vi "Lab14_LabView.vi"() -> ()   [LabVIEW 2022 SP3]
uses:
  <vilib>/Instr/_visa.llb/VISA Configure Serial Port (Instr).vi
panel:
  out "POTENCIOMETRO 8":dbl(knob) scale=0.0..1023.0
  out "POTENCIOMETRO 7":dbl(knob) scale=0.0..1023.0
  out "POTENCIOMETRO 6":dbl(knob) scale=0.0..1023.0
  out "POTENCIOMETRO 5":dbl(knob) scale=0.0..1023.0
  out "POTENCIOMETRO 4":dbl(knob) scale=0.0..1023.0
  out "POTENCIOMETRO 3":dbl(knob) scale=0.0..1023.0
  out "POTENCIOMETRO 2":dbl(knob) scale=0.0..1023.0
  out "POTENCIOMETRO":i32(knob) scale=0.0..1023.0
  in  "VISA resource name":refnum<visa-resource-name>
  in  "stop":bool
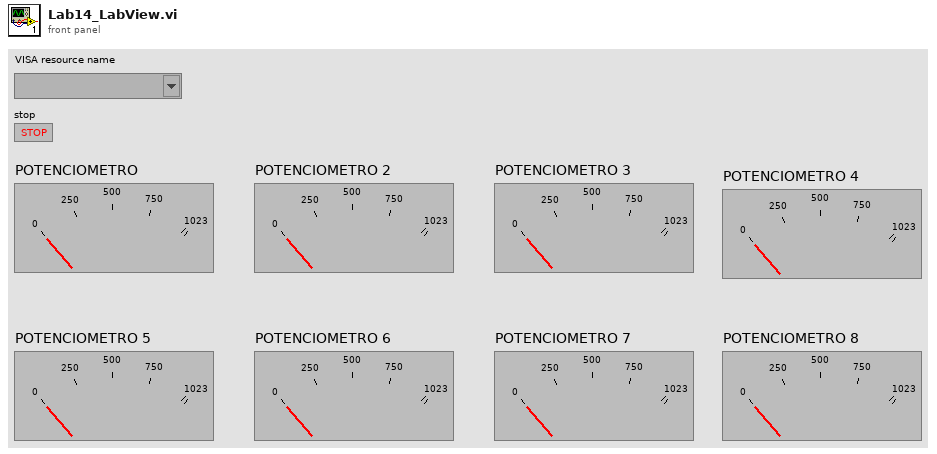
[diagram p1: front panel]
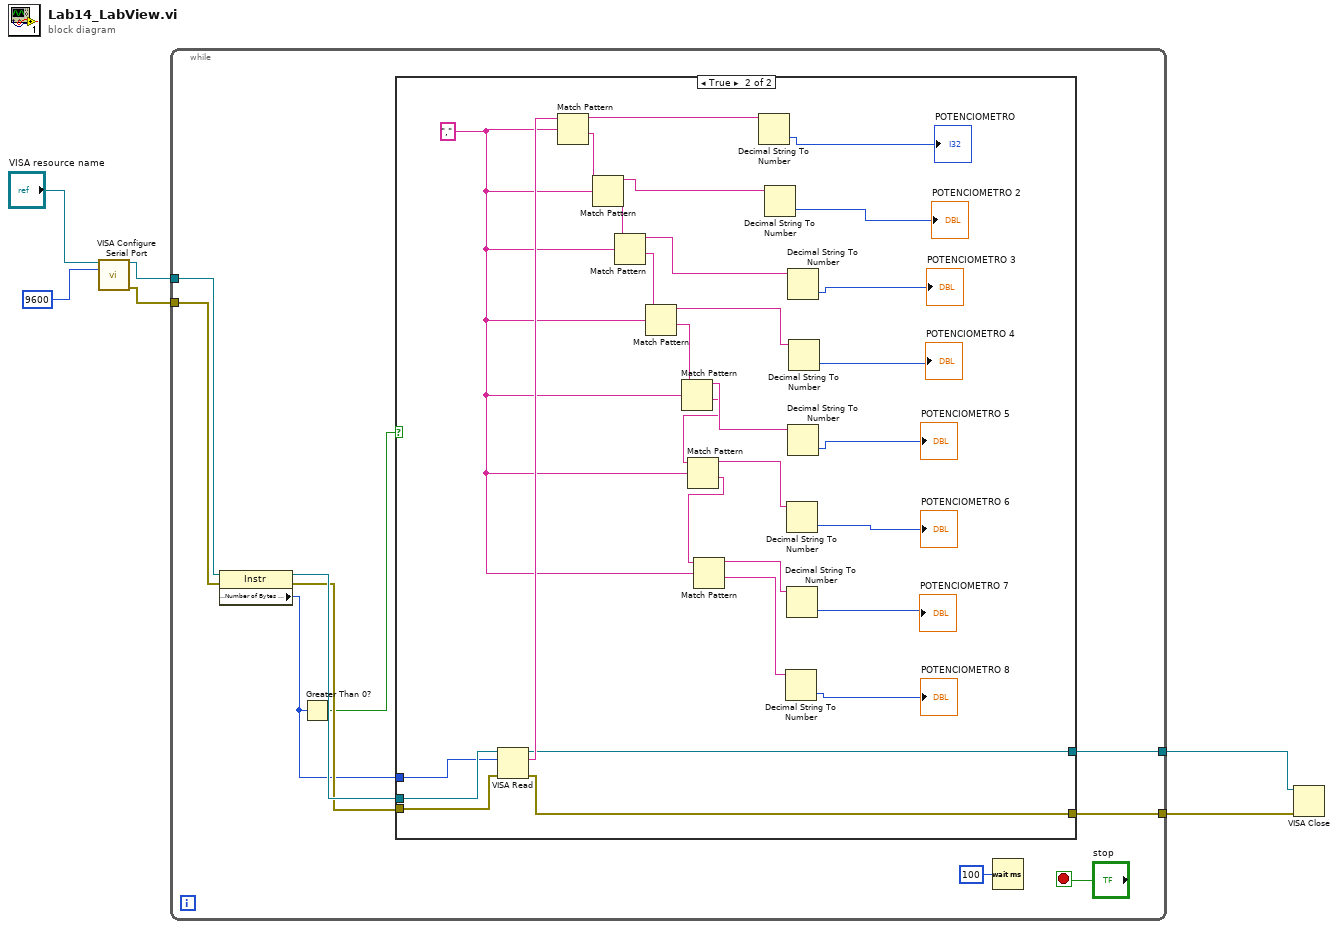
[diagram p0: block diagram]
diagram:
  n1 = call-poly "VISA Configure Serial Port"("VISA resource name"="VISA resource name", "baud rate (9600)"=u32 9600) -> ("VISA resource name out"=w6:refnum<visa-resource-name>, "error out"=w5:errorcluster)  [unwired: 12 in]
  n2 = while {
    tunnel: w6 -> [w10]
    tunnel: w5 -> [w9]
    tunnel: [w8] -> w2
    tunnel: [w7] -> w1
    stop <- "stop" stop-if-true
    n3 = property class="Instr"(reference=w10, error in=w9) -> (reference out=w14:refnum<visa-resource-name>, error out=w13:errorcluster, "Serial Settings:Number of Bytes at Serial Port"=w11:u32)
    n4 = Greater Than 0?(x=w11) -> (x > 0?=w12:bool)
    n5 = case shown="True" w12 {
      tunnel: w14 -> [w18 w47]
      tunnel: w13 -> [w17 w46]
      tunnel: w11 -> [_ w45]
      tunnel: [w17 w20] -> w8
      tunnel: [w18 w19] -> w7
      frame False {
      }
      frame True {
        w26 = ","
        n6 = VISA Read(VISA resource name=w47, byte count=w45, error in (no error)=w46) -> (VISA resource name out=w19:refnum<visa-resource-name>, read buffer=w44:string, error out=w20:errorcluster)  [unwired: 1 out]
        n7 = Match Pattern(string=w44, regular expression=w26) -> (before substring=w43:string, after substring=w42:string)  [unwired: 1 in, 2 out]
        n8 = Match Pattern(string=w42, regular expression=w26) -> (before substring=w41:string, after substring=w40:string)  [unwired: 1 in, 2 out]
        n9 = Match Pattern(string=w40, regular expression=w26) -> (before substring=w39:string, after substring=w38:string)  [unwired: 1 in, 2 out]
        n10 = Match Pattern(string=w38, regular expression=w26) -> (before substring=w36:string, after substring=w37:string)  [unwired: 1 in, 2 out]
        n11 = Match Pattern(string=w37, regular expression=w26) -> (before substring=w35:string, after substring=w25:string)  [unwired: 1 in, 2 out]
        n12 = Match Pattern(string=w25, regular expression=w26) -> (before substring=w23:string, after substring=w24:string)  [unwired: 1 in, 2 out]
        n13 = Match Pattern(string=w24, regular expression=w26) -> (before substring=w22:string, after substring=w21:string)  [unwired: 1 in, 2 out]
        n14 = Decimal String To Number(string=w43) -> (number=→"POTENCIOMETRO":i32)  [unwired: 2 in, 1 out]
        n15 = Decimal String To Number(string=w41) -> (number=→"POTENCIOMETRO 2":i32)  [unwired: 2 in, 1 out]
        n16 = Decimal String To Number(string=w21) -> (number=→"POTENCIOMETRO 8":i32)  [unwired: 2 in, 1 out]
        n17 = Decimal String To Number(string=w23) -> (number=→"POTENCIOMETRO 6":i32)  [unwired: 2 in, 1 out]
        n18 = Decimal String To Number(string=w22) -> (number=→"POTENCIOMETRO 7":i32)  [unwired: 2 in, 1 out]
        n19 = Decimal String To Number(string=w39) -> (number=→"POTENCIOMETRO 3":i32)  [unwired: 2 in, 1 out]
        n20 = Decimal String To Number(string=w35) -> (number=→"POTENCIOMETRO 5":i32)  [unwired: 2 in, 1 out]
        n21 = Decimal String To Number(string=w36) -> (number=→"POTENCIOMETRO 4":i32)  [unwired: 2 in, 1 out]
      }
    }
    n22 = Wait (ms)(milliseconds to wait=u32 100) -> ()  [unwired: 1 out]
  }
  n23 = VISA Close(VISA resource name=w1, error in (no error)=w2) -> ()  [unwired: 1 out]
